vi "getSerializedData.vi"(0 "reference":refnum<class "InitialStateNode.lvclass">, 5 "error in (no error)":errorcluster) -> (14 "reference out":refnum<class "InitialStateNode.lvclass">, 15 "parent":refnum<class "AbstractNode.lvclass">, 16 "children":refnum<class "AbstractNode.lvclass">[](array[class]), 17 "xmlOut":string, 19 "error out":errorcluster)   [LabVIEW 2016, in "InitialStateNode.lvclass"]
doc: "getSerializedData"
uses:
  <resource>/Framework/Providers/Open_GDS/UML/InitialStateNode_class/InitialStateNode.lvclass
  C:/Program Files (x86)/National Instruments/LabVIEW 2016/resource/Framework/Providers/Open_GDS/UML/RectangularNode_class/RectangularNode.lvclass
  C:/Program Files (x86)/National Instruments/LabVIEW 2016/resource/Framework/Providers/Open_GDS/UML/AbstractNode_class/AbstractNode.lvclass
  <resource>/Framework/Providers/Open_GDS/UML/AbstractNode_class/AbstractNode.lvclass
  <resource>/Framework/Providers/Open_GDS/UML/General/Rectangle/Rectangle Rectangle2D.ctl
  <resource>/Framework/Providers/Open_GDS/UML/MultiLineString_class/MultiLineString.lvclass
  <resource>/Framework/Providers/Open_GDS/UML/RectangularNode_class/RectangularNode.lvclass
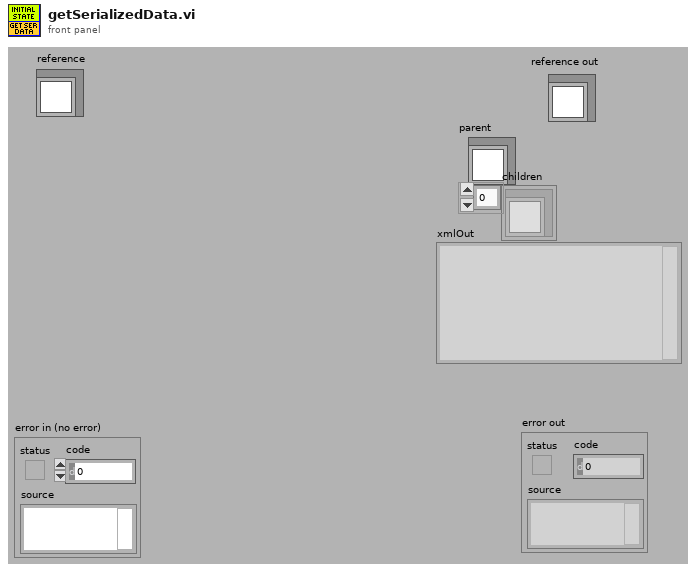
[diagram p1: front panel]
types:
  T1 = typedef "Rectangle Rectangle2D.ctl" = cluster{"x":dbl, "y":dbl, "width":dbl, "height":dbl}
  T2 = cluster{"Base class":cluster{"Base class":cluster{"parent":refnum<k1>, "children":refnum<k1>[]}, "bounds":T1}, "name":refnum<k1>, "DEFAULT_WIDTH":i32, "DEFAULT_HEIGHT":i32}
  T3 = typedef "InitialStateNode.lvclass/ObjectAttributes.ctl" = cluster{"name":refnum<class "MultiLineString.lvclass">, "DEFAULT_WIDTH":i32, "DEFAULT_HEIGHT":i32}
  T4 = typedef "RectangularNode.lvclass/ObjectAttributes.ctl" = cluster{"bounds":T1}
  T5 = typedef "AbstractNode.lvclass/ObjectAttributes.ctl" = cluster{"parent":refnum<class "AbstractNode.lvclass">, "children":refnum<class "AbstractNode.lvclass">[], "Hidden":bool}
  T6 = cluster{"Attributes":cluster{"Base class":cluster{"Base class":cluster{"parent":refnum<k1>, "children":refnum<k1>[]}, "bounds":T1}, "name":refnum<k1>, "DEFAULT_WIDTH":i32, "DEFAULT_HEIGHT":i32}, "text":string}
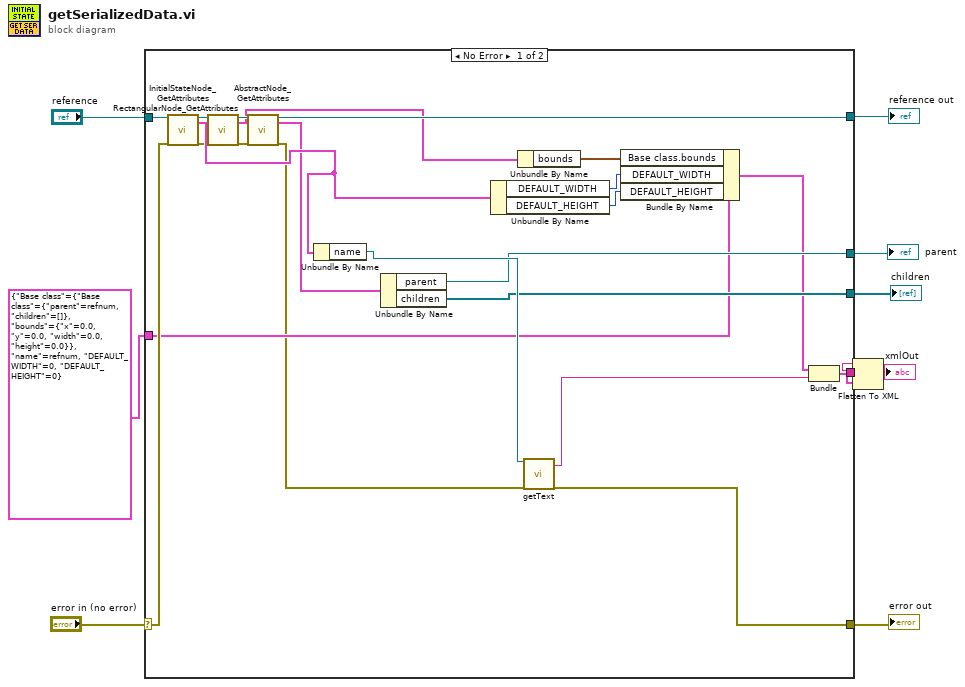
[diagram p0: block diagram]
diagram:
  n1 = case shown="No Error" "error in (no error)" {
    selector: "error in (no error)" -> [w31 w32]
    tunnel: "reference" -> [w30 w33]
    tunnel: [w23 w32] -> w6
    tunnel: [w11 w33] -> w5
    tunnel: [w26 _] -> w4
    tunnel: [w25 _] -> w3
    tunnel: [w24 _] -> w2
    tunnel: T2 {"Base class"={"Base class"={"parent"=refnum, "children"=[]}, "bounds"={"x"=0.0, "y"=0.0, "width"=0.0, "height"=0.0}}, "name"=refnum, "DEFAULT_WIDTH"=0, "DEFAULT_HEIGHT"=0} ("Attributes") -> [w19 _]
    frame No Error {
      n2 = call <resource>:"InitialStateNode_GetAttributes.vi"("reference in"=w30, "error in (no error)"=w31) -> ("reference out"=w16:refnum<class "InitialStateNode.lvclass">, "Data"=w17:T3, "error out"=w15:errorcluster)  [unwired: 1 in, 14 out]
      n3 = call <resource>:"RectangularNode_GetAttributes.vi"("reference in"=w16, "error in (no error)"=w15) -> ("reference out"=w14:refnum<class "InitialStateNode.lvclass">, "Data"=w10:T4, "error out"=w13:errorcluster)  [unwired: 14 in, 1 out]
      n4 = call <resource>:"AbstractNode_GetAttributes.vi"("reference in"=w14, "error in (no error)"=w13) -> ("reference out"=w11:refnum<class "InitialStateNode.lvclass">, "Data"=w9:T5, "error out"=w12:errorcluster)  [unwired: 14 in, 1 out]
      n5 = Unbundle By Name(w17) -> ("name"=w28:refnum<class "MultiLineString.lvclass">)
      n6 = Unbundle By Name(w9) -> ("parent"=w26:refnum<class "AbstractNode.lvclass">, "children"=w25:refnum<class "AbstractNode.lvclass">[])
      n7 = Unbundle By Name(w17) -> ("DEFAULT_WIDTH"=w21:i32, "DEFAULT_HEIGHT"=w20:i32)
      n8 = Unbundle By Name(w10) -> ("bounds"=w22:T1)
      n9 = call-dynamic "getText.vi"("reference"=w28, "error in (no error)"=w12) -> ("text"=w27:string, "error out"=w23:errorcluster)  [unwired: 16 out]
      n10 = Bundle By Name(cluster=w19, "Base class.bounds"=w22, "DEFAULT_WIDTH"=w21, "DEFAULT_HEIGHT"=w20) -> (w18:T2)
      n11 = Bundle("Attributes"=w18, "text"=w27) -> (w29:T6)  [unwired: 1 out]
      n12 = Flatten To XML(anything=w29) -> (xml string=w24:string)
    }
    frame Error {
    }
  }
  "reference out" <- w5
  "error out" <- w6
  "parent" <- w4
  "children" <- w3
  "xmlOut" <- w2
